vi "Start Stream.vi"(1 "Auto-Advance":bool, 5 "Injection Countdown":bool, 8 "error in (no error)":errorcluster, 10 "Camera Settings":T1={"Exposure Time (ms)"=100.0, "Binning"=enum."2x2", "Scan Mode"=0, "Frames to Acquire"=1000.0, "Pixel Correction"=FALSE, "Frames to Skip"=0, "File Path"=path "", "Duty cycle"=0.0, "ALEX"=FALSE, "Shutter Enable"=[]} {"Exposure Time (ms)" min=1.0 max=10000.0 step=1.0}, 11 "Application in":refnum<class "Application.lvclass">) -> (0 "error out":errorcluster, 3 "Application out":refnum<class "Application.lvclass">)   [LabVIEW 2018, in "Application.lvlib" / "Application.lvclass"]
uses:
  Application.lvclass
  C:/Program Files/National Instruments/LabVIEW 2018/vi.lib/ActorFramework/Actor/Actor.lvclass
  Resources/Type Defs/Camera Settings.ctl
  User Interface/Progress Window/Progress Window.lvclass
  User Interface/Countdown Timer/Countdown Timer.lvclass
  C:/LVCUR/flash-gordon/User Interface/UI Window/UI Window.lvclass
  Application.lvclass/Application.ctl
  Hardware/Synchronization Device Messages/Set All Msg/Set All Msg.lvclass/Set All Msg.ctl
  <vilib>/ActorFramework/Message Enqueuer/Message Enqueuer.lvclass/Message Enqueuer.ctl
  <vilib>/ActorFramework/Message Enqueuer/Enqueue.vi
  Hardware/Synchronization Device Messages/Set All Msg/Set All Msg.lvclass
  C:/Program Files/National Instruments/LabVIEW 2018/vi.lib/ActorFramework/Message/Message.lvclass
  <vilib>/ActorFramework/Message Priority Queue/Priority Enqueue.vi
  Resources/GLOBAL/GLOBAL Time-critical.vi
  <vilib>/ActorFramework/Actor/Actor.lvclass
panel:
  in  "Auto-Infuse":bool
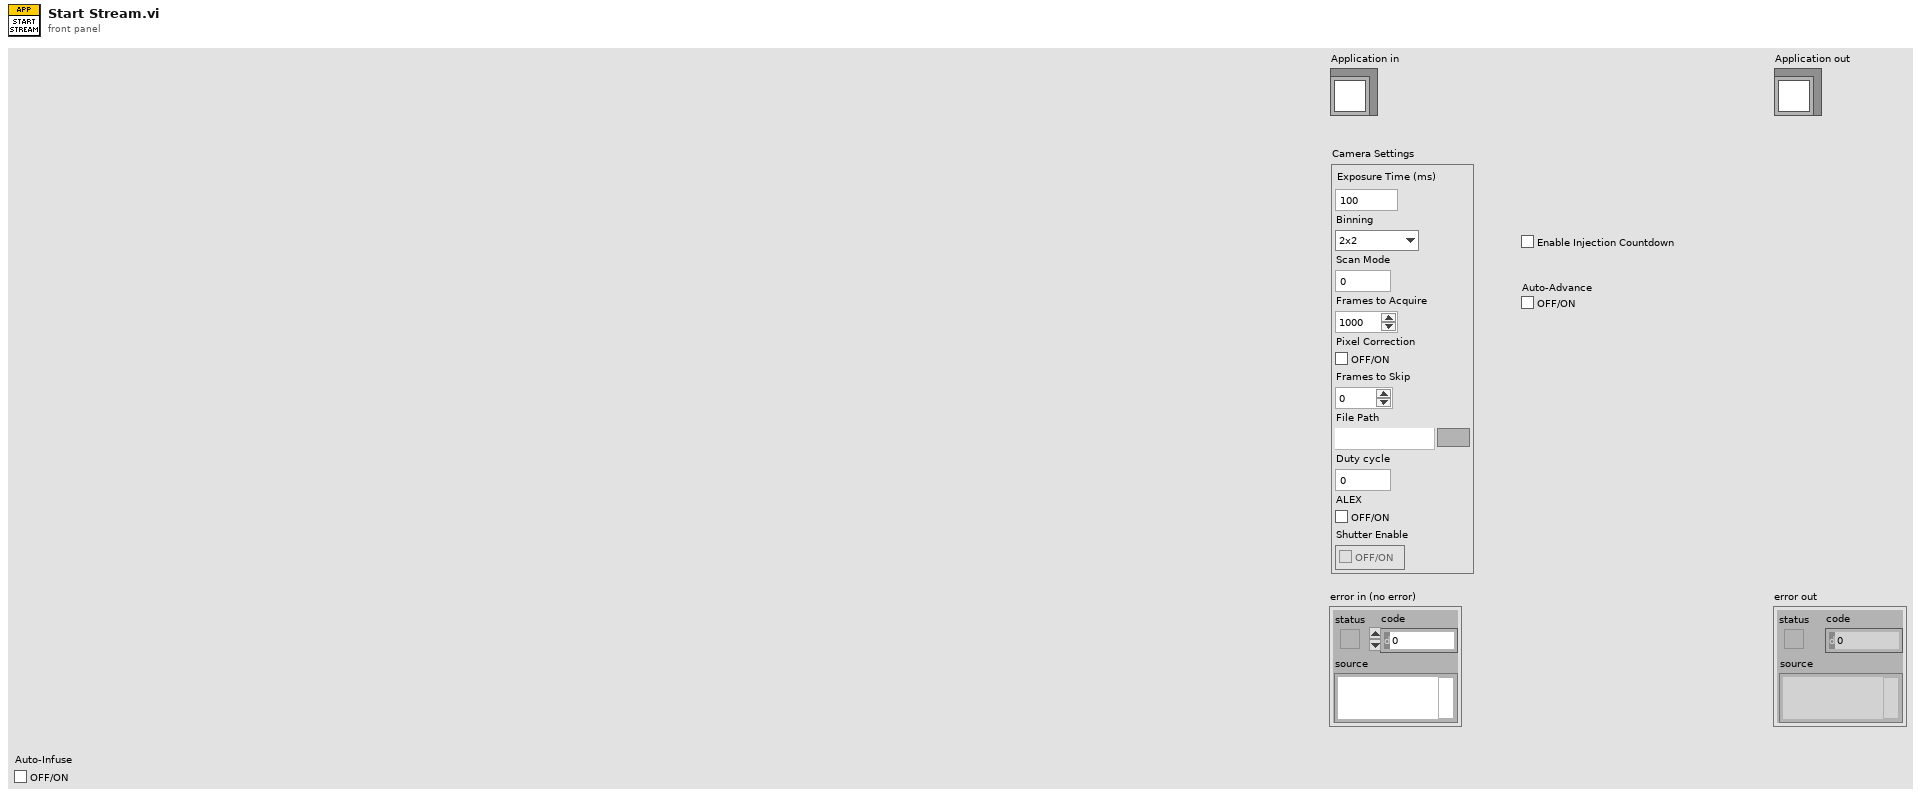
[diagram p1: front panel]
types:
  T1 = typedef "Camera Settings.ctl" = cluster{"Exposure Time (ms)":dbl, "Binning":enum16{"1x1", "2x2", "4x4"}, "Scan Mode":i32, "Frames to Acquire":dbl, "Pixel Correction":bool, "Frames to Skip":u32, "File Path":path, "Duty cycle":dbl, "ALEX":bool, "Shutter Enable":bool[]}
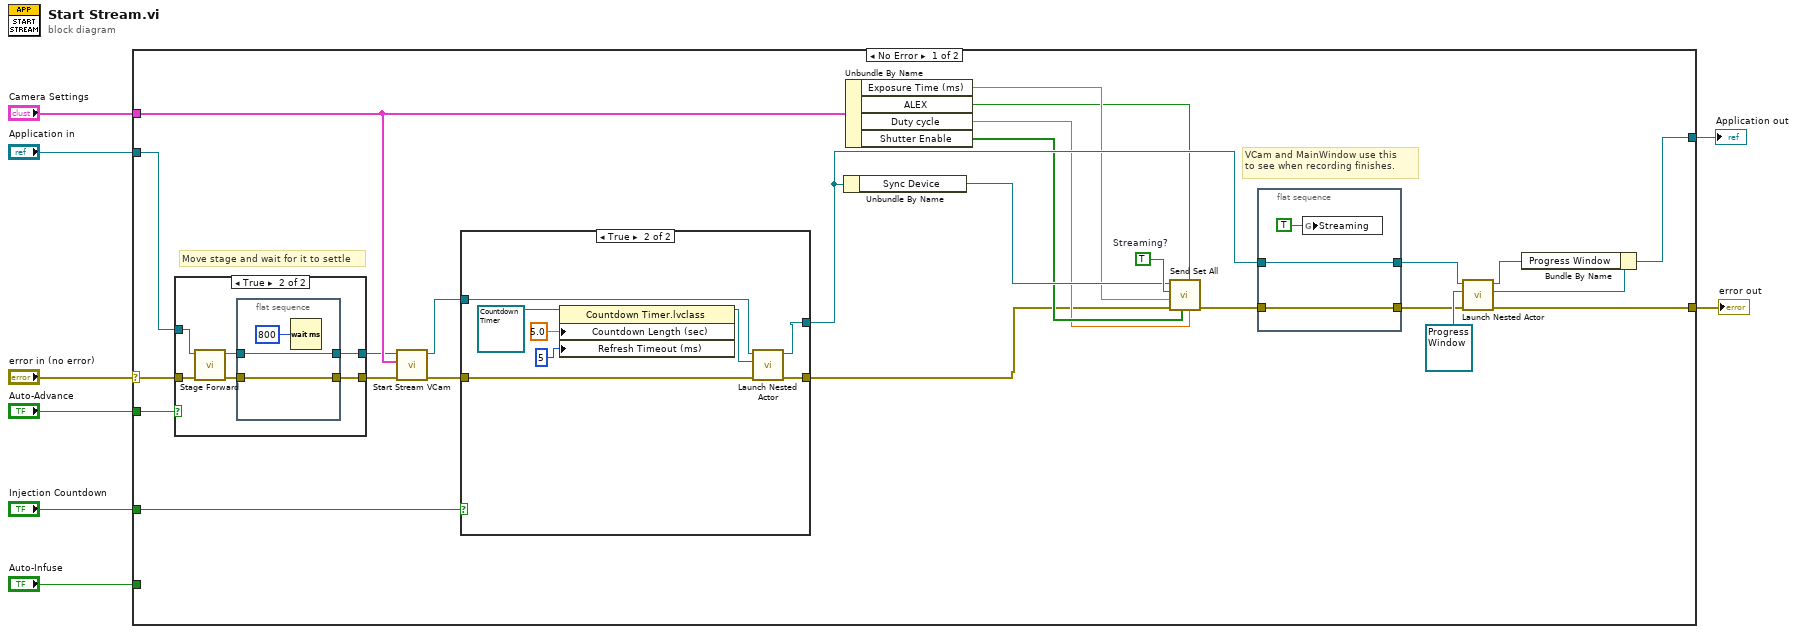
[diagram p0: block diagram]
diagram:
  n1 = case shown="No Error" "error in (no error)" {
    selector: "error in (no error)" -> [w28 w59]
    tunnel: [w32 w59] -> w7
    tunnel: "Application in" -> [w29 w58]
    tunnel: "Camera Settings" -> [w22 _]
    tunnel: "Injection Countdown" -> [w26 _]
    tunnel: "Auto-Advance" -> [w27 _]
    tunnel: [w24 w58] -> w2
    tunnel: "Auto-Infuse" -> [_ _]
    frame No Error {
      w18 = TRUE  # Streaming?
      # "Move stage and wait for it to settle"
      # "VCam and MainWindow use this\nto see when recording finishes."
      n2 = case shown="True" w27 {
        tunnel: w29 -> [w38 w44]
        tunnel: w28 -> [w37 w43]
        tunnel: [w38 w41] -> w10
        tunnel: [w37 w39] -> w9
        frame False {
        }
        frame True {
          n3 = call-dynamic "Stage Forward.vi"("error in (no error)"=w43, "Application in"=w44) -> ("error out"=w40:errorcluster, "Application out"=w42:refnum<class "Application.lvclass">)  [unwired: 8 in]
          n4 = flat-sequence {
            tunnel: [w46] -> w41
            tunnel: w42 -> [w46]
            tunnel: w40 -> [w45]
            tunnel: [w45] -> w39
            frame #0 {
              n5 = Wait (ms)(milliseconds to wait=u32 800) -> ()  [unwired: 1 out]
            }
          }
        }
      }
      n6 = call "Start Stream VCam.vi"("error in (no error)"=w9, "Camera Settings"=w22, "Application in"=w10) -> ("error out"=w21:errorcluster, "Application out"=w20:refnum<class "Application.lvclass">)  [unwired: 7 in]
      n7 = case shown="True" w26 {
        tunnel: w20 -> [w49 w55]
        tunnel: [w49 w57] -> w19
        tunnel: w21 -> [w48 w56]
        tunnel: [w48 w50] -> w11
        frame False {
        }
        frame True {
          n8 = property class="Countdown Timer.lvclass"(reference=refnum<class "Countdown Timer.lvclass"> refnum ("Countdown Timer.lvlib:Countdown Timer.lvclass"), "Countdown Length (sec)"=5.0, "Refresh Timeout (ms)"=5) -> (reference out=w51:refnum<class "Countdown Timer.lvclass">)  [unwired: 1 in, 1 out]
          n9 = call <vilib>:"Launch Nested Actor.vi"("error in (no error)"=w56, "Nested Actor"=w51, "Caller Actor in"=w55) -> ("error out"=w50:errorcluster, "Caller Actor out"=w57:refnum<class "Application.lvclass">)  [unwired: 6 in, 1 out]
        }
      }
      n10 = Unbundle By Name(w19) -> ("Sync Device"=w16:refnum<class "Message Enqueuer.lvclass">)
      n11 = Unbundle By Name(w22) -> ("Exposure Time (ms)"=w15:dbl, "ALEX"=w14:bool, "Duty cycle"=w12:dbl, "Shutter Enable"=w13:bool[])
      n12 = call "Send Set All.vi"("Duty Cycle"=w12, "ALEX?"=w14, "Shutter Enable"=w13, "error in (no error)"=w11, "Interval (ms)"=w15, "Streaming?"=w18, "Message Enqueuer"=w16) -> ("error out"=w17:errorcluster)  [unwired: 3 in, 1 out]
      n13 = flat-sequence {
        tunnel: w17 -> [w35]
        tunnel: [w35] -> w25
        tunnel: w19 -> [w34]
        tunnel: [w34] -> w23
        frame #0 {
          n14 = global write "GLOBAL Time-critical.vi" "Streaming"(TRUE ("Streaming")) -> ()
        }
      }
      n15 = call <vilib>:"Launch Nested Actor.vi"("error in (no error)"=w25, "Nested Actor"=refnum<class "Progress Window.lvclass"> refnum ("Progress Window.lvlib:Progress Window.lvclass"), "Caller Actor in"=w23) -> ("error out"=w32:errorcluster, "Nested Actor's Enqueuer"=w30:refnum<class "Message Enqueuer.lvclass">, "Caller Actor out"=w31:refnum<class "Application.lvclass">)  [unwired: 6 in]
      n16 = Bundle By Name(cluster=w31, "Progress Window"=w30) -> (w24:refnum<class "Application.lvclass">)
    }
    frame Error {
    }
  }
  "error out" <- w7
  "Application out" <- w2
